vi "Exercise4.7-FM_RTL-SDR_RX - Event.vi"() -> ()   [LabVIEW 2013]
uses:
  <vilib>/sound2/lvsound2.llb/Sampling Mode.ctl
  <vilib>/sound2/lvsound2.llb/Sound Data Format.ctl
  <vilib>/sound2/lvsound2.llb/Sound Output Write (DBL Single).vi
  <instrlib>/rtlsdr/rtlsdr.lvlib
panel:
  out "error out 4":errorcluster
  out "error out 3":errorcluster
  out "error out 2":errorcluster
  in  "Volume":dbl(knob)=0.8 min=0.0 max=2.0 step=0.1 scale=0.0..2.0
  in  "Sample Rate":dbl=256000.0
  out "EXIT":bool=TRUE
  in  "FM  Frequency":dbl(slide)=92700000.0 min=85000000.0 max=108000000.0 step=50000.0 scale=85000000.0..108000000.0 scale format="%#_6p"
  in  "Device index":u32=1
  out "Samples Acquired":u32
  out "DevRefnum":u64
  in  "stop":bool
  out "error out":errorcluster
  out "FM Spectrum":cluster{dbl[], dbl[]}[](graph)
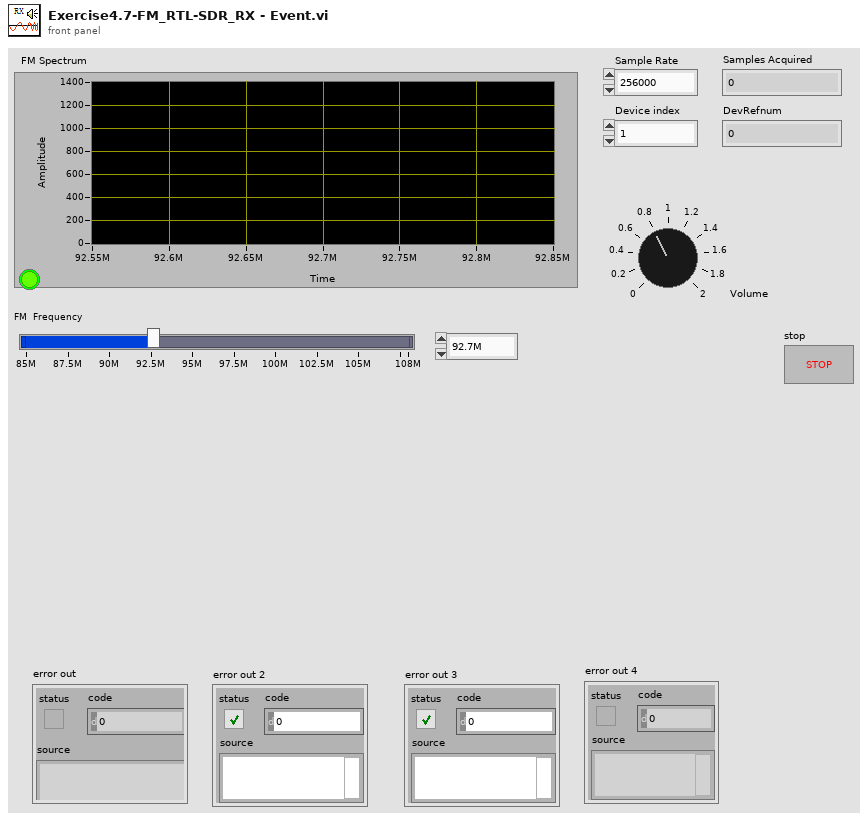
[diagram p1: front panel]
types:
  T1 = typedef "Sound Data Format.ctl" = cluster{"sample rate (S/s)":dbl, "number of channels":i32, "bits per sample":i32}
  T2 = typedef "Sampling Mode.ctl" = i32
  T3 = typedef "Sound Output Task ID.ctl" = u32
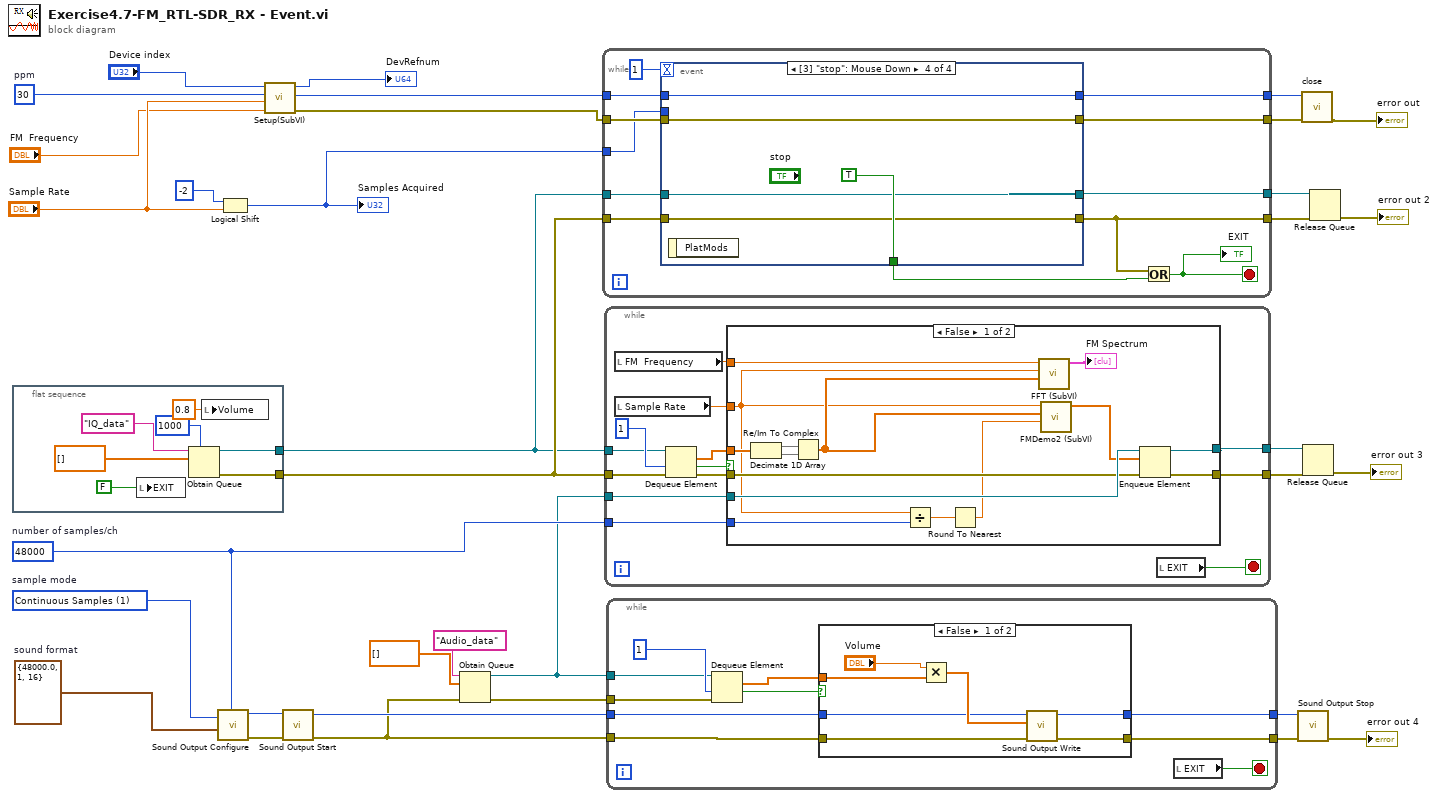
[diagram p0: block diagram]
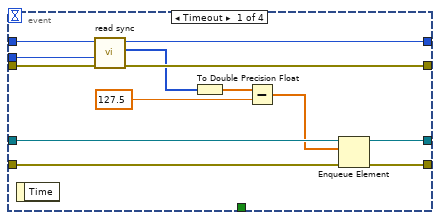
[diagram p4: hidden frame]
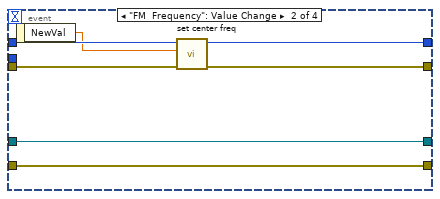
[diagram p5: hidden frame]
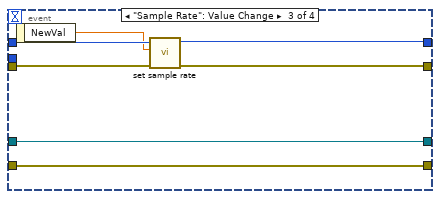
[diagram p6: hidden frame]
diagram:
  w17 = 30  # ppm
  w25 = T1 {"sample rate (S/s)"=48000.0, "number of channels"=1, "bits per sample"=16}  # sound format
  w12 = 48000  # number of samples/ch
  w22 = T2 1 items=["Finite Samples", "Continuous Samples"]  # sample mode
  n1 = flat-sequence {
    tunnel: [w39] -> w13
    tunnel: [w36] -> w14
    frame #0 {
      n2 = local write "EXIT"(FALSE ("EXIT")) -> ()
      n3 = Obtain Queue(max queue size (-1, unlimited)=1000, name (unnamed)="IQ_data", element data type=dbl[] [] ("samples")) -> (queue out=w39:refnum<queue>, error out=w36:errorcluster)  [unwired: 2 in, 1 out]
      n4 = local write "Volume"(0.8 ("Volume")) -> ()
    }
  }
  n5 = call <vilib>:"Sound Output Configure.vi"("number of samples/ch"=w12, "sample mode"=w22, "sound format"=w25) -> ("error out"=w23:errorcluster, "task ID"=w24:T3)  [unwired: 7 in]
  n6 = Logical Shift(y=i16 -2, x="Sample Rate") -> (x << y=w26:u32)
  "Samples Acquired" <- w26
  n7 = call "Setup(SubVI).vi"("FM  Frequency"="FM  Frequency", "IQ Rate"="Sample Rate", "ppm"=w17, "Device index"="Device index") -> ("error out"=w31:errorcluster, "DevRefnum"=w32:u64, "DevRefnum 2"=→"DevRefnum":u64)  [unwired: 5 in]
  n8 = call <vilib>:"Sound Output Start.vi"("error in (no error)"=w23, "task ID"=w24) -> ("error out"=w4:errorcluster, "task ID out"=w7:T3)  [unwired: 8 in]
  n9 = Obtain Queue(name (unnamed)="Audio_data", element data type=dbl[] [] ("Decimated Array"), error in (no error)=w4) -> (queue out=w6:refnum<queue>, error out=w5:errorcluster)  [unwired: 2 in, 1 out]
  n10 = while {
    tunnel: [w51] -> w29
    tunnel: w32 -> [w53]
    tunnel: w31 -> [w52]
    tunnel: [w50] -> w28
    tunnel: w26 -> [w45]
    tunnel: w13 -> [w49]
    tunnel: [w48] -> w18
    tunnel: w14 -> [w47]
    tunnel: [w46] -> w15
    stop <- w44 stop-if-true
    n11 = event shown="[3] \"stop\": Mouse Down" {
      selector: _ -> [_ _ _ _]
      dyn-events: _ -> [_ _ _ _]
      timeout: 1 -> [_ _ _ _]
      tunnel: w53 -> [w66 w73 w80 w82]
      tunnel: w52 -> [w65 w70 w78 w81]
      tunnel: [w64 w72 w79 w82] -> w51
      tunnel: [w63 w71 w76 w81] -> w50
      tunnel: w49 -> [w62 w68 w75 w84]
      tunnel: [w61 w68 w75 w84] -> w48
      tunnel: w47 -> [w60 w67 w74 w83]
      tunnel: [w59 w67 w74 w83] -> w46
      tunnel: w45 -> [w58 _ _ _]
      tunnel: [_ _ _ TRUE] -> w42
      event Timeout {
        n12 = event-data() -> ()  [unwired: 1 in, 1 out]
        n13 = call <instrlib>:"read sync.vi"("error in (no error)"=w65, "len"=w58, "DevRefnum"=w66) -> ("error out"=w63:errorcluster, "buf 2"=w55:u8[], "DevRefnum"=w64:u64)  [unwired: 6 in]
        n14 = To Double Precision Float(number=w55) -> (double precision float=w56:dbl[])
        n15 = Subtract(x=w56, y=127.5) -> (x-y=w54:dbl[])
        n16 = Enqueue Element(queue=w62, element=w54, error in (no error)=w60) -> (queue out=w61:refnum<queue>, error out=w59:errorcluster)  [unwired: 1 in, 1 out]
      }
      event "FM  Frequency": Value Change {
        n17 = event-data() -> ("NewVal"=w69:dbl)  [unwired: 1 in]
        n18 = call <instrlib>:"set center freq.vi"("error in (no error)"=w70, "freq"=w69, "DevRefnum"=w73) -> ("error out"=w71:errorcluster, "DevRefnum"=w72:u64)  [unwired: 6 in, 1 out]
      }
      event "Sample Rate": Value Change {
        n19 = event-data() -> ("NewVal"=w77:dbl)  [unwired: 1 in]
        n20 = call <instrlib>:"set sample rate.vi"("error in (no error)"=w78, "rate"=w77, "DevRefnum"=w80) -> ("error out"=w76:errorcluster, "DevRefnum"=w79:u64)  [unwired: 6 in, 1 out]
      }
      event "stop": Mouse Down {
        n21 = event-data() -> ()  [unwired: 1 in, 1 out]
      }
    }
    n22 = Or(x=w46, y=w42) -> (x .or. y?=w44:bool)
    "EXIT" <- w44
  }
  n23 = while {
    tunnel: w14 -> [w91]
    tunnel: w13 -> [w90]
    tunnel: w6 -> [w89]
    tunnel: w12 -> [w88]
    tunnel: [w87] -> w11
    tunnel: [w86] -> w10
    stop <- w98 stop-if-true
    n24 = local read "FM  Frequency"() -> (w95:dbl)
    n25 = local read "Sample Rate"() -> (w96:dbl)
    n26 = Dequeue Element(queue=w90, timeout in ms (-1)=1, error in (no error)=w91) -> (element=w93:dbl[], timed out?=w92:bool, error out=w94:errorcluster)  [unwired: 1 out]
    n27 = case shown="False" w92 {
      tunnel: w93 -> [w113 _]
      tunnel: w96 -> [w100 _]
      tunnel: w89 -> [w110 w115]
      tunnel: [w109 w115] -> w87
      tunnel: [w108 w114] -> w86
      tunnel: w94 -> [w107 w114]
      tunnel: w95 -> [w104 _]
      tunnel: w88 -> [w102 _]
      frame False {
        n28 = Decimate 1D Array(w113) -> (w112:dbl[], w111:dbl[])
        n29 = Re/Im To Complex(1:w111, 2:w112) -> (0:w105:cdb[])
        n30 = Divide(x=w100, y=w102) -> (x/y=w103:dbl)
        n31 = Round To Nearest(number=w103) -> (nearest integer value=w101:dbl)
        n32 = call "FFT (SubVI).vi"("Array"=w105, "Sample Rate"=w100, "FM  Frequency"=w104) -> ("FM Spectrum"=→"FM Spectrum":cluster{dbl[], dbl[]}[])  [unwired: 8 in]
        n33 = call "FMDemo2 (SubVI).vi"("Numeric"=w101, "Array"=w105, "Sample Rate"=w100) -> ("Decimated Array"=w106:dbl[])  [unwired: 8 in]
        n34 = Enqueue Element(queue=w110, element=w106, error in (no error)=w107) -> (queue out=w109:refnum<queue>, error out=w108:errorcluster)  [unwired: 1 in, 1 out]
      }
      frame True {
      }
    }
    n35 = local read "EXIT"() -> (w98:bool)
  }
  n36 = while {
    tunnel: [w121] -> w9
    tunnel: [w120] -> w8
    tunnel: w7 -> [w119]
    tunnel: w6 -> [w118]
    tunnel: w5 -> [w117]
    tunnel: w4 -> [w116]
    stop <- w125 stop-if-true
    n37 = Dequeue Element(queue=w118, timeout in ms (-1)=1, error in (no error)=w117) -> (element=w123:dbl[], timed out?=w122:bool)  [unwired: 2 out]
    n38 = case shown="False" w122 {
      tunnel: w123 -> [w128 _]
      tunnel: w116 -> [w132 w133]
      tunnel: [w131 w133] -> w120
      tunnel: [w130 _] -> w121
      tunnel: w119 -> [w126 _]
      frame False {
        n39 = Multiply(x="Volume", y=w128) -> (x*y=w129:dbl[])
        n40 = call-poly <vilib>:"Sound Output Write.vi"("error in (no error)"=w132, "data"=w129, "task ID"=w126) -> ("error out"=w131:errorcluster, "task ID out"=w130:T3)  [unwired: 7 in]
      }
      frame True {
      }
    }
    n41 = local read "EXIT"() -> (w125:bool)
  }
  n42 = call <vilib>:"Sound Output Stop.vi"("error in (no error)"=w8, "task ID"=w9) -> ("error out"=→"error out 4":errorcluster)  [unwired: 8 in, 1 out]
  n43 = call <instrlib>:"close.vi"("error in (no error)"=w28, "DevRefnum"=w29) -> ("error out"=→"error out":errorcluster)  [unwired: 8 in, 1 out]
  n44 = Release Queue(queue=w11, error in (no error)=w10) -> (error out=→"error out 3":errorcluster)  [unwired: 1 in, 2 out]
  n45 = Release Queue(queue=w18, error in (no error)=w15) -> (error out=→"error out 2":errorcluster)  [unwired: 1 in, 2 out]
